vi "Latch.vi"(8 "reset?":bool, 10 "default_value":bool, 11 "value_to_latch":bool) -> (2 "Output":bool)   [LabVIEW 2020]
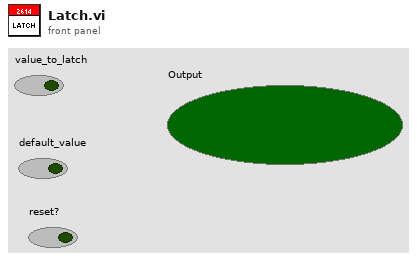
[diagram p1: front panel]
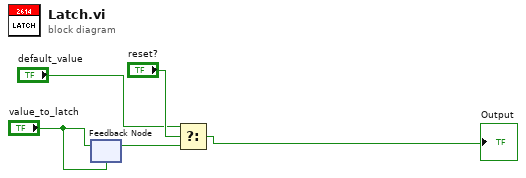
[diagram p0: block diagram]
diagram:
  n1 = feedback-in #1("value_to_latch") -> ()
  n2 = feedback #1("value_to_latch") -> (w1:bool)
  n3 = Select(t="default_value", s="reset?", f=w1) -> (s? t:f=→"Output":bool)
